vi "Read Paths.vi"(8 "error in (no error)":errorcluster, 11 "Setting Database in":refnum<class "Setting Database.lvclass">) -> (0 "error out":errorcluster, 2 "Paths":refnum<class "Path Settings.lvclass">[](array[class]), 3 "Setting Database out":refnum<class "Setting Database.lvclass">)   [LabVIEW 2019, in "Setting Database.lvclass"]
uses:
  Setting Database.lvclass
  Path Settings/Path Settings.lvclass
  Setting Database.lvclass/Setting Database.ctl
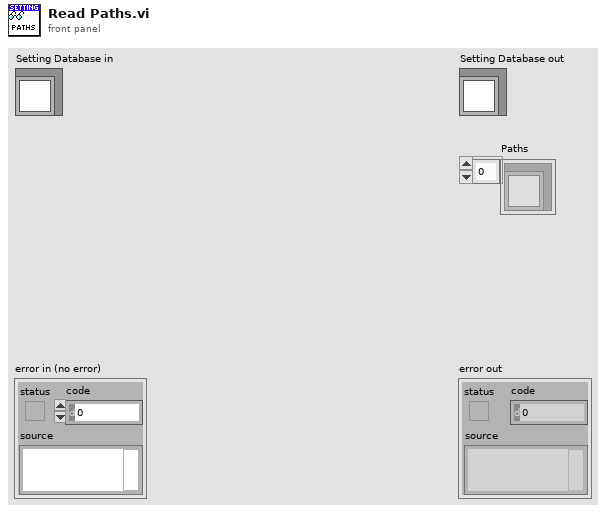
[diagram p1: front panel]
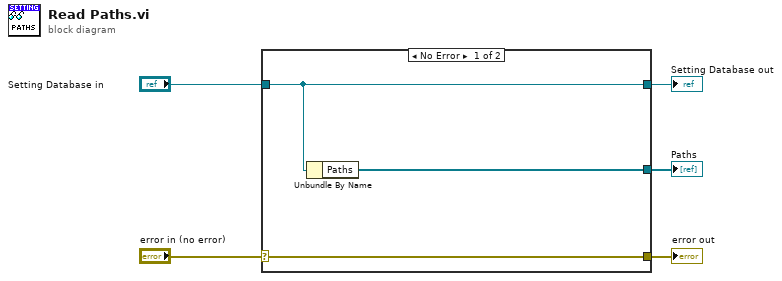
[diagram p0: block diagram]
diagram:
  n1 = case shown="No Error" "error in (no error)" {
    selector: "error in (no error)" -> [w8 w9]
    tunnel: [w8 w9] -> w4
    tunnel: [w7 w10] -> w2
    tunnel: "Setting Database in" -> [w7 w10]
    tunnel: [w6 _] -> w1
    frame No Error {
      n2 = Unbundle By Name(w7) -> ("Paths"=w6:refnum<class "Path Settings.lvclass">[])
    }
    frame Error {
    }
  }
  "error out" <- w4
  "Setting Database out" <- w2
  "Paths" <- w1
